vi "Variant to String.vi"(8 "error in (no error)":errorcluster, 11 "Data (Variant)":variant) -> (0 "error out":errorcluster, 3 "Value":string)   [LabVIEW 2016, in "Data.lvclass"]
uses:
  Data.lvclass
  <vilib>/Utility/error.llb/Error Cluster From Error Code.vi
  <vilib>/ErrorRing/Error Ring.xnode
  <vilib>/Utility/Data Type/NI_Data Type.lvlib
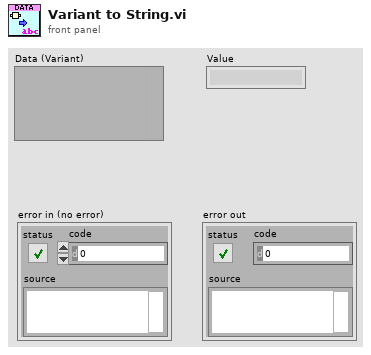
[diagram p1: front panel]
types:
  T1 = typedef "NI_Data Type.lvlib/Data Type.ctl" = enum8{"Invalid Type", "Void", "I8", "I16", "I32", "I64", "U8", "U16", "U32", "U64", "Single Float", "Double Float", "Extended Float", "Single Complex", "Double Complex", "Extended Complex", "Enum U8", "Enum U16", "Enum U32", "Enum U64", "Single Float With Unit", "Double Float With Unit", "Extended Float With Unit", "Single Complex with Unit", "Double Complex with Unit", "Extended Complex with Unit", "Boolean", "String", "Path", "Picture", "Tag", "Array", "Cluster", "Variant", "LV Variant", "Waveform", "Timestamp", "Digital Waveform", "Digital Data", "ExpressData", "Refnum", "External Data", "VI", "Poly VI", "LabVIEW Class Instance", "Fixed Point"}
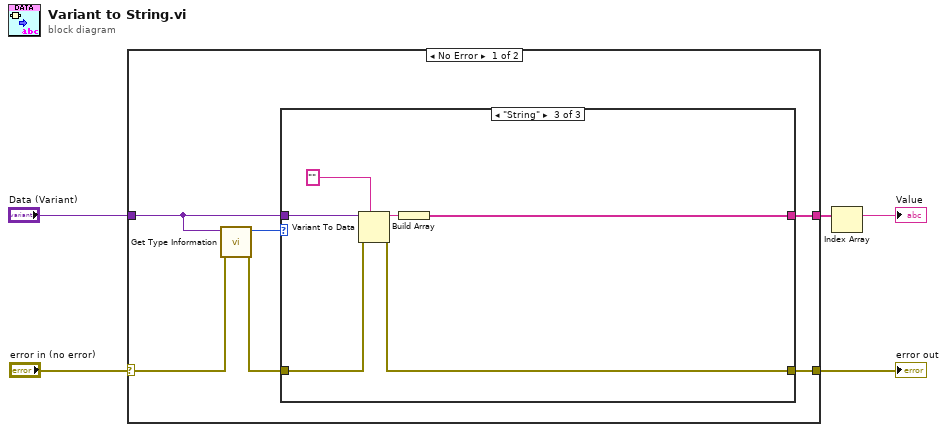
[diagram p0: block diagram]
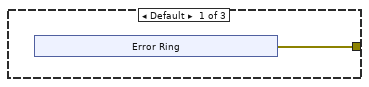
[diagram p2: hidden frame]
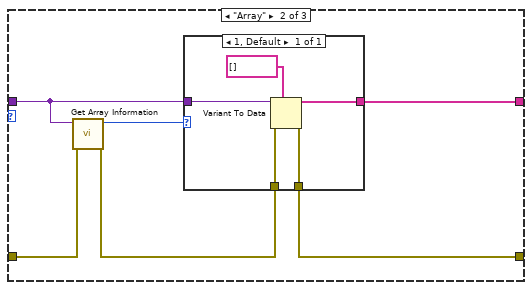
[diagram p3: hidden frame]
diagram:
  n1 = case shown="No Error" "error in (no error)" {
    selector: "error in (no error)" -> [w6 w34]
    tunnel: [w10 _] -> w2
    tunnel: [w7 w34] -> w5
    tunnel: "Data (Variant)" -> [w9 _]
    frame No Error {
      n2 = call <vilib>:"Get Type Information.vi"("error in (no error)"=w6, "Variant"=w9) -> ("error out"=w8:errorcluster, "Type"=w11:T1)  [unwired: 5 in, 3 out]
      n3 = case shown="\"String\"" w11 {
        tunnel: [w12 w22 w29] -> w7
        tunnel: [_ w17 w31] -> w10
        tunnel: w9 -> [_ w21 w32]
        tunnel: w8 -> [_ w20 w30]
        frame Default {
          n4 = xnode "Error Ring"() -> ("error out"=w12:errorcluster)
        }
        frame "Array" {
          n5 = call <vilib>:"Get Array Information.vi"("error in (no error)"=w20, "Variant"=w21) -> ("error out"=w19:errorcluster, "Number of Dimensions"=w18:i32)  [unwired: 6 in, 2 out]
          n6 = case shown="1, Default" w18 {
            tunnel: [w26] -> w22
            tunnel: w21 -> [w25]
            tunnel: w19 -> [w24]
            tunnel: [w23] -> w17
            frame 1, Default {
              n7 = Variant To Data(error in=w24, type=string[] [], Variant=w25) -> (data=w23:string[], error out=w26:errorcluster)
            }
          }
        }
        frame "String" {
          n8 = Variant To Data(error in=w30, type="", Variant=w32) -> (data=w33:string, error out=w29:errorcluster)
          n9 = Build Array(w33) -> (w31:string[])
        }
      }
    }
    frame Error {
    }
  }
  "error out" <- w5
  n10 = Index Array(array=w2) -> (element=→"Value":string)  [unwired: 1 in]
